vi "filter_calcs.vi"(8 "Detector 3 Correlations In":T1, 9 "Detector 1 Correlations In":T1, 10 "Detector 3":i16, 11 "Detector 1":i16) -> (0 "Detector 3 Correlations Out":T1, 1 "Detector 1 Correlations Out":T1)   [LabVIEW 2015]
uses:
  Detector_Cluster.ctl
  <vilib>/rvi/Emulation/niFpgaEmulationIsFPGAContextNoSignature.vi
  <vilib>/rvi/Emulation/niFpgaSctlEmulationGetInTimedLoop.vi
  <vilib>/rvi/errors/niFpgaSetErrorForExecOnDevCompSimple.vi
  <vilib>/rvi/eio/common/nirviEmuReportErrorAndStop.vi
  <vilib>/rvi/DataTransferAndStorage/Container/Common/niFpgaContainerGetUniqueNameForEmu.vi
  <vilib>/rvi/FIFO/Fifo_Resource/nirvififoEmulationSetSize.vi
  <vilib>/rvi/FIFO/Fifo_Resource/nirviFifoEmulationQueueMgr.vi
  <instcachedir>/0/nirviFifoEmulationQueueMgr_E5CAEC123FF24DC58D834DCA3CDAA9B5.lvgen/nirviFifoEmulationQueueMgr_E5CAEC123FF24DC58D834DCA3CDAA9B5_002.vi
  <vilib>/rvi/FIFO/Fifo_Resource/nirvififoEmulationDetermineInputValidOut.vi
  <vilib>/rvi/FIFO/Fifo_Resource/nirvififoEmulationCreateLock.vi
  <vilib>/rvi/Emulation/niFpgaProcessEmulError.vi
  <vilib>/rvi/FIFO/Fifo_Resource/nirvififoEmulationObtainLock.vi
  <vilib>/rvi/FIFO/Fifo_Resource/nirvififoEmulationReleaseLock.vi
  <vilib>/rvi/occurrence/nirviWaitOnOccurrenceBase.vi
  <vilib>/rvi/errors/nirviReportUnexpectedCaseInternalError.vi
  <vilib>/rvi/errors/nirviReportUnexpectedCaseInternalError (U32).vi
  <vilib>/rvi/DataTransferAndStorage/Container/Common/niFpgaContainerExecOnDevCompGetState.vi
  <vilib>/Utility/error.llb/Clear Errors.vi
  <vilib>/rvi/interface/RandomDataEmulation/niFpgaRandomDataHandleErrors.vi
  <vilib>/rvi/DataTransferAndStorage/Container/XNode/niFpgaContainer.xnode
  <vilib>/rvi/FIFO/Fifo_Resource/nirvififoEmulationWrite.vi
  <vilib>/rvi/FIFO/Fifo_Resource/niFpgaFifoEmulationRefIn.vi
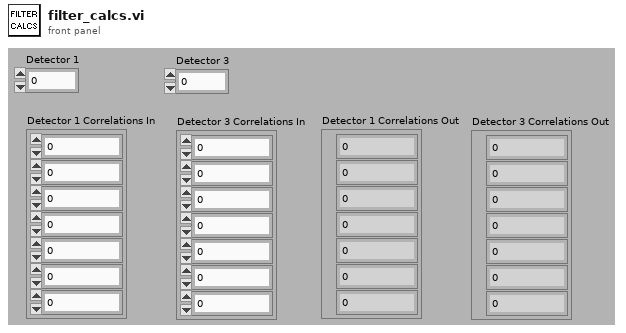
[diagram p1: front panel]
types:
  T1 = typedef "Detector_Cluster.ctl" = cluster{"1":i32, "2":i32, "3":i32, "4":i32, "5":i32, "6":i32, "7":i32}
  T2 = cluster{"Average Out":i32, "Next State":u16, "Detector 1 Correlation out":i32, "Detector 3 Correlation out":i32, "Velocity Count out":i32, "Detector counter out":i32, "Timeout count out":u32}
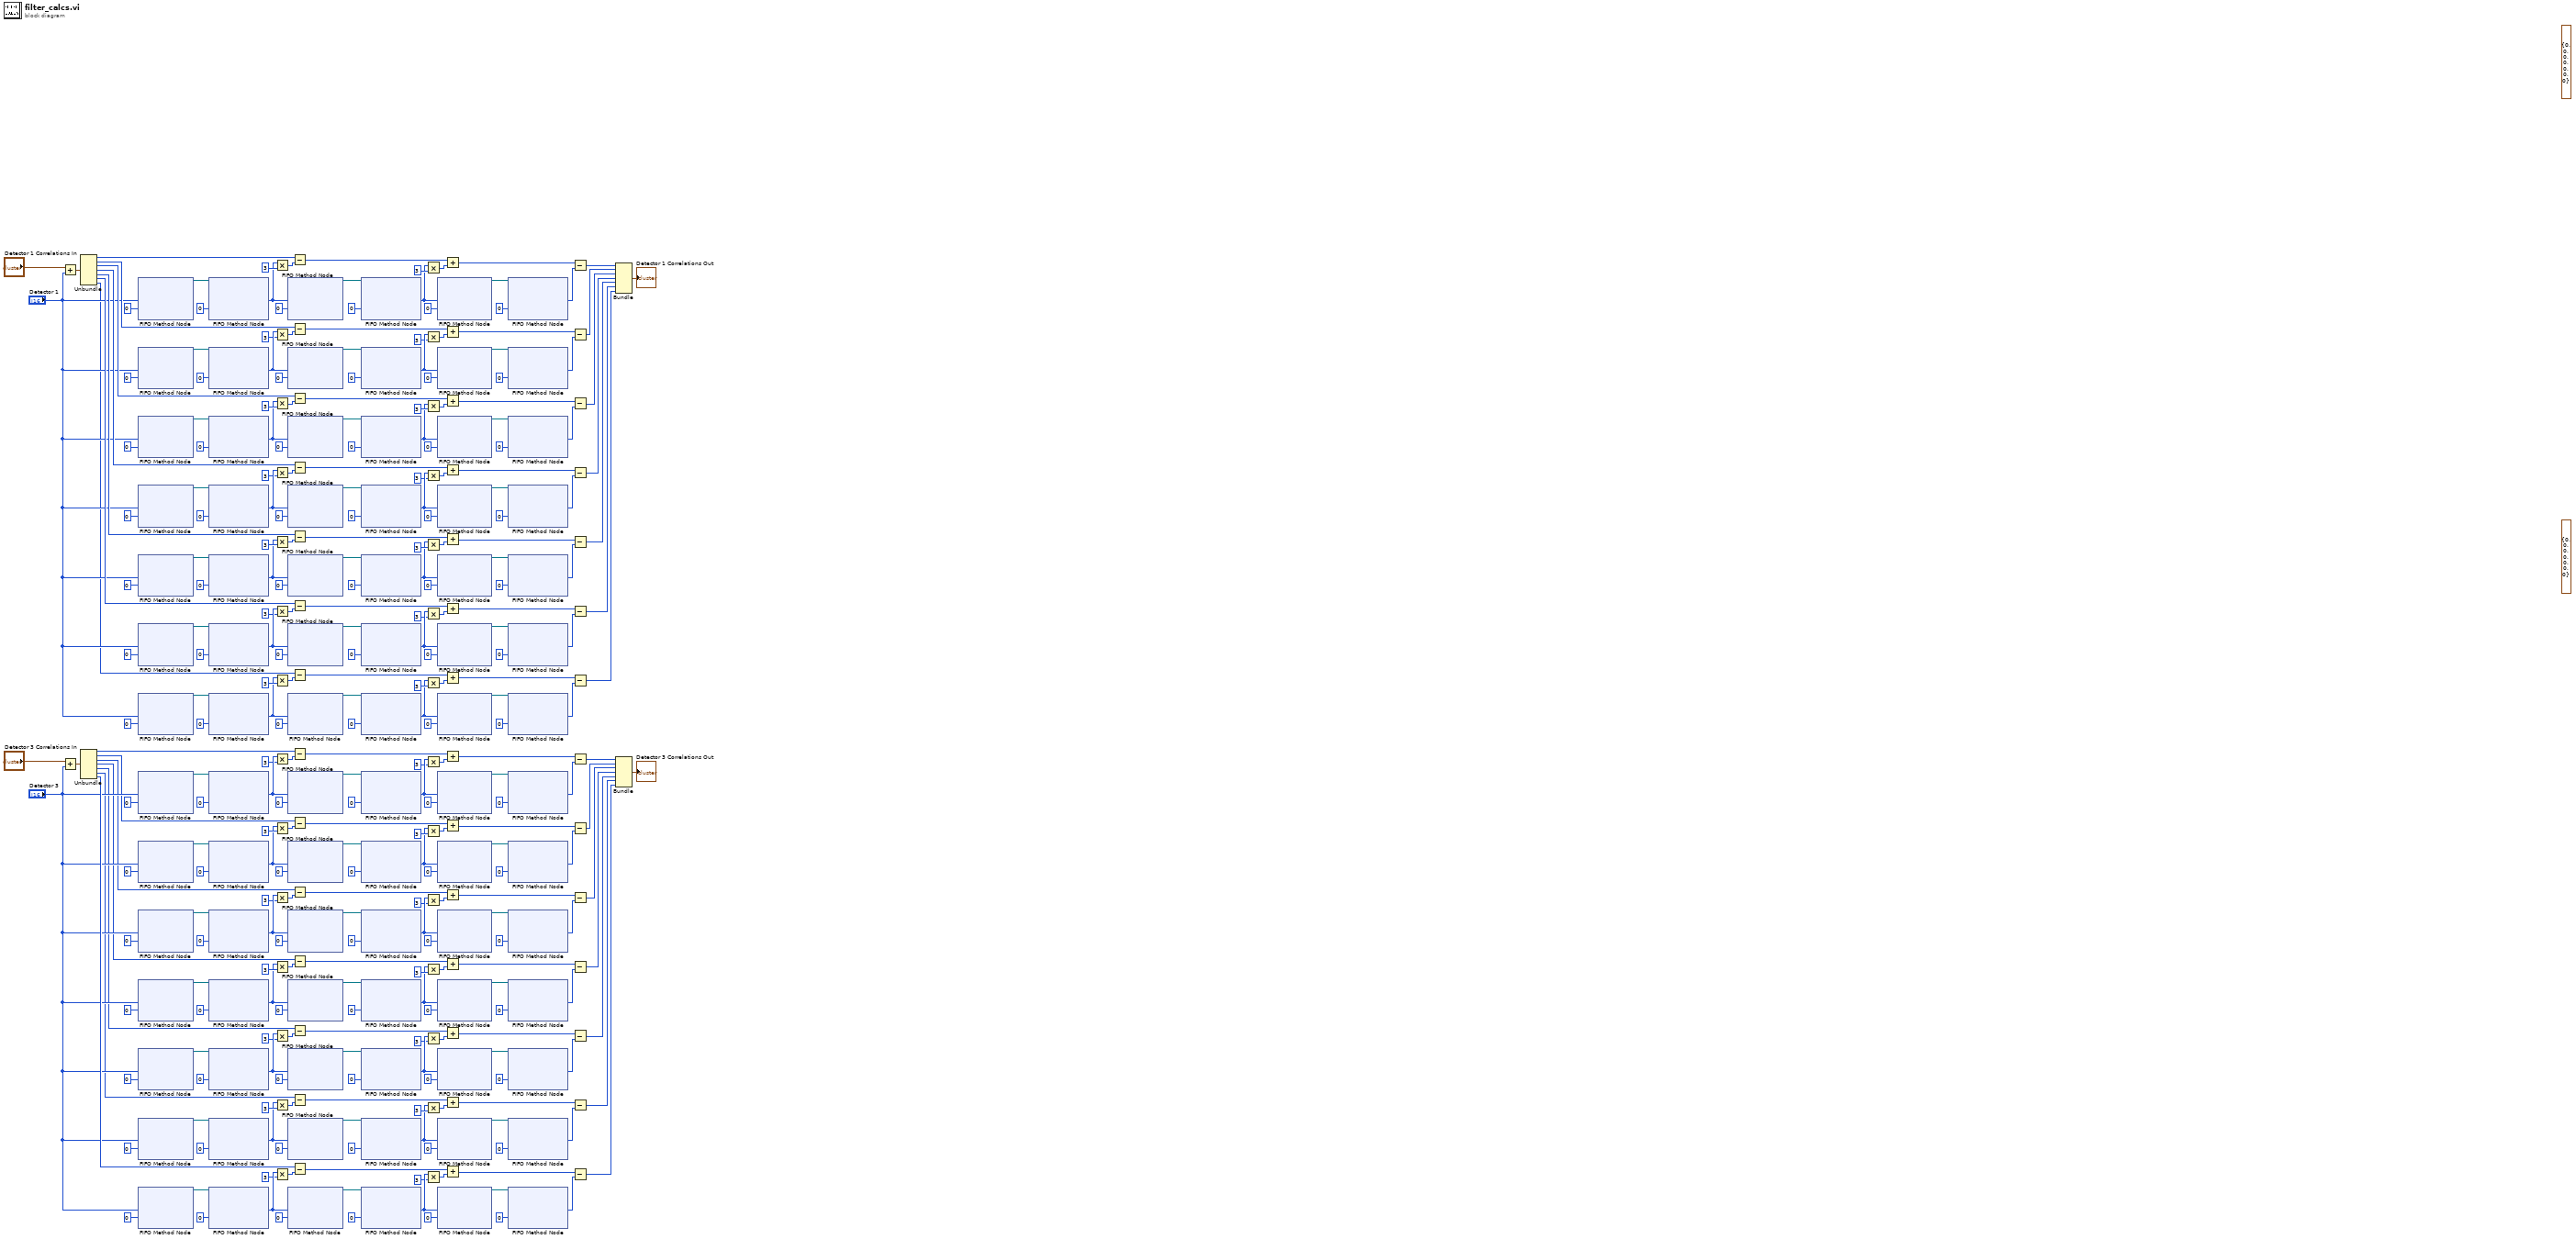
[diagram p0: block diagram]
diagram:
  (unwired) T2 {"Average Out"=0, "Next State"=0, "Detector 1 Correlation out"=0, "Detector 3 Correlation out"=0, "Velocity Count out"=0, "Detector counter out"=0, "Timeout count out"=0} ("Output Cluster")
  (unwired) T2 {"Average Out"=0, "Next State"=0, "Detector 1 Correlation out"=0, "Detector 3 Correlation out"=0, "Velocity Count out"=0, "Detector counter out"=0, "Timeout count out"=0} ("Output Cluster")
  n1 = Add(x="Detector 1 Correlations In", y="Detector 1") -> (x+y=w275:T1)
  n2 = Add(x="Detector 3 Correlations In", y="Detector 3") -> (x+y=w14:T1)
  n3 = Unbundle(w275) -> ("1"=w273:i32, "2"=w247:i32, "3"=w226:i32, "4"=w207:i32, "5"=w187:i32, "6"=w167:i32, "7"=w146:i32)
  n4 = Unbundle(w14) -> ("1"=w16:i32, "2"=w42:i32, "3"=w63:i32, "4"=w82:i32, "5"=w102:i32, "6"=w122:i32, "7"=w143:i32)
  n5 = xnode ("FIFO Method Node")("Element"="Detector 1", "Timeout"=0) -> ("FIFO Out"=w278:refnum<k21>)  [unwired: 1 in, 1 out]
  n6 = xnode ("FIFO Method Node")("Element"="Detector 1", "Timeout"=0) -> ("FIFO Out"=w258:refnum<k21>)  [unwired: 1 in, 1 out]
  n7 = xnode ("FIFO Method Node")("Element"="Detector 1", "Timeout"=0) -> ("FIFO Out"=w235:refnum<k21>)  [unwired: 1 in, 1 out]
  n8 = xnode ("FIFO Method Node")("Element"="Detector 1", "Timeout"=0) -> ("FIFO Out"=w218:refnum<k21>)  [unwired: 1 in, 1 out]
  n9 = xnode ("FIFO Method Node")("Element"="Detector 1", "Timeout"=0) -> ("FIFO Out"=w195:refnum<k21>)  [unwired: 1 in, 1 out]
  n10 = xnode ("FIFO Method Node")("Element"="Detector 1", "Timeout"=0) -> ("FIFO Out"=w178:refnum<k21>)  [unwired: 1 in, 1 out]
  n11 = xnode ("FIFO Method Node")("Element"="Detector 1", "Timeout"=0) -> ("FIFO Out"=w155:refnum<k21>)  [unwired: 1 in, 1 out]
  n12 = xnode ("FIFO Method Node")("Element"="Detector 3", "Timeout"=0) -> ("FIFO Out"=w11:refnum<k21>)  [unwired: 1 in, 1 out]
  n13 = xnode ("FIFO Method Node")("Element"="Detector 3", "Timeout"=0) -> ("FIFO Out"=w31:refnum<k21>)  [unwired: 1 in, 1 out]
  n14 = xnode ("FIFO Method Node")("Element"="Detector 3", "Timeout"=0) -> ("FIFO Out"=w54:refnum<k21>)  [unwired: 1 in, 1 out]
  n15 = xnode ("FIFO Method Node")("Element"="Detector 3", "Timeout"=0) -> ("FIFO Out"=w71:refnum<k21>)  [unwired: 1 in, 1 out]
  n16 = xnode ("FIFO Method Node")("Element"="Detector 3", "Timeout"=0) -> ("FIFO Out"=w94:refnum<k21>)  [unwired: 1 in, 1 out]
  n17 = xnode ("FIFO Method Node")("Element"="Detector 3", "Timeout"=0) -> ("FIFO Out"=w111:refnum<k21>)  [unwired: 1 in, 1 out]
  n18 = xnode ("FIFO Method Node")("Element"="Detector 3", "Timeout"=0) -> ("FIFO Out"=w134:refnum<k21>)  [unwired: 1 in, 1 out]
  n19 = xnode ("FIFO Method Node")("Timeout"=0, "FIFO In"=w278) -> ("Element"=w284:i16)  [unwired: 2 out]
  n20 = xnode ("FIFO Method Node")("Timeout"=0, "FIFO In"=w258) -> ("Element"=w252:i16)  [unwired: 2 out]
  n21 = xnode ("FIFO Method Node")("Timeout"=0, "FIFO In"=w235) -> ("Element"=w241:i16)  [unwired: 2 out]
  n22 = xnode ("FIFO Method Node")("Timeout"=0, "FIFO In"=w218) -> ("Element"=w212:i16)  [unwired: 2 out]
  n23 = xnode ("FIFO Method Node")("Timeout"=0, "FIFO In"=w195) -> ("Element"=w201:i16)  [unwired: 2 out]
  n24 = xnode ("FIFO Method Node")("Timeout"=0, "FIFO In"=w178) -> ("Element"=w172:i16)  [unwired: 2 out]
  n25 = xnode ("FIFO Method Node")("Timeout"=0, "FIFO In"=w155) -> ("Element"=w161:i16)  [unwired: 2 out]
  n26 = xnode ("FIFO Method Node")("Timeout"=0, "FIFO In"=w11) -> ("Element"=w5:i16)  [unwired: 2 out]
  n27 = xnode ("FIFO Method Node")("Timeout"=0, "FIFO In"=w31) -> ("Element"=w37:i16)  [unwired: 2 out]
  n28 = xnode ("FIFO Method Node")("Timeout"=0, "FIFO In"=w54) -> ("Element"=w48:i16)  [unwired: 2 out]
  n29 = xnode ("FIFO Method Node")("Timeout"=0, "FIFO In"=w71) -> ("Element"=w77:i16)  [unwired: 2 out]
  n30 = xnode ("FIFO Method Node")("Timeout"=0, "FIFO In"=w94) -> ("Element"=w88:i16)  [unwired: 2 out]
  n31 = xnode ("FIFO Method Node")("Timeout"=0, "FIFO In"=w111) -> ("Element"=w117:i16)  [unwired: 2 out]
  n32 = xnode ("FIFO Method Node")("Timeout"=0, "FIFO In"=w134) -> ("Element"=w128:i16)  [unwired: 2 out]
  n33 = Multiply(x=w284, y=i16 3) -> (x*y=w274:i16)
  n34 = Multiply(x=w252, y=i16 3) -> (x*y=w261:i16)
  n35 = Multiply(x=w241, y=i16 3) -> (x*y=w232:i16)
  n36 = Multiply(x=w212, y=i16 3) -> (x*y=w221:i16)
  n37 = Multiply(x=w201, y=i16 3) -> (x*y=w192:i16)
  n38 = Multiply(x=w172, y=i16 3) -> (x*y=w181:i16)
  n39 = Multiply(x=w161, y=i16 3) -> (x*y=w152:i16)
  n40 = Multiply(x=w5, y=i16 3) -> (x*y=w15:i16)
  n41 = Multiply(x=w37, y=i16 3) -> (x*y=w28:i16)
  n42 = Multiply(x=w48, y=i16 3) -> (x*y=w57:i16)
  n43 = Multiply(x=w77, y=i16 3) -> (x*y=w68:i16)
  n44 = Multiply(x=w88, y=i16 3) -> (x*y=w97:i16)
  n45 = Multiply(x=w117, y=i16 3) -> (x*y=w108:i16)
  n46 = Multiply(x=w128, y=i16 3) -> (x*y=w137:i16)
  n47 = xnode ("FIFO Method Node")("Element"=w284, "Timeout"=0) -> ("FIFO Out"=w277:refnum<k21>)  [unwired: 1 in, 1 out]
  n48 = xnode ("FIFO Method Node")("Element"=w252, "Timeout"=0) -> ("FIFO Out"=w259:refnum<k21>)  [unwired: 1 in, 1 out]
  n49 = xnode ("FIFO Method Node")("Element"=w241, "Timeout"=0) -> ("FIFO Out"=w234:refnum<k21>)  [unwired: 1 in, 1 out]
  n50 = xnode ("FIFO Method Node")("Element"=w212, "Timeout"=0) -> ("FIFO Out"=w219:refnum<k21>)  [unwired: 1 in, 1 out]
  n51 = xnode ("FIFO Method Node")("Element"=w201, "Timeout"=0) -> ("FIFO Out"=w194:refnum<k21>)  [unwired: 1 in, 1 out]
  n52 = xnode ("FIFO Method Node")("Element"=w172, "Timeout"=0) -> ("FIFO Out"=w179:refnum<k21>)  [unwired: 1 in, 1 out]
  n53 = xnode ("FIFO Method Node")("Element"=w161, "Timeout"=0) -> ("FIFO Out"=w154:refnum<k21>)  [unwired: 1 in, 1 out]
  n54 = xnode ("FIFO Method Node")("Element"=w5, "Timeout"=0) -> ("FIFO Out"=w12:refnum<k21>)  [unwired: 1 in, 1 out]
  n55 = xnode ("FIFO Method Node")("Element"=w37, "Timeout"=0) -> ("FIFO Out"=w30:refnum<k21>)  [unwired: 1 in, 1 out]
  n56 = xnode ("FIFO Method Node")("Element"=w48, "Timeout"=0) -> ("FIFO Out"=w55:refnum<k21>)  [unwired: 1 in, 1 out]
  n57 = xnode ("FIFO Method Node")("Element"=w77, "Timeout"=0) -> ("FIFO Out"=w70:refnum<k21>)  [unwired: 1 in, 1 out]
  n58 = xnode ("FIFO Method Node")("Element"=w88, "Timeout"=0) -> ("FIFO Out"=w95:refnum<k21>)  [unwired: 1 in, 1 out]
  n59 = xnode ("FIFO Method Node")("Element"=w117, "Timeout"=0) -> ("FIFO Out"=w110:refnum<k21>)  [unwired: 1 in, 1 out]
  n60 = xnode ("FIFO Method Node")("Element"=w128, "Timeout"=0) -> ("FIFO Out"=w135:refnum<k21>)  [unwired: 1 in, 1 out]
  n61 = Subtract(x=w273, y=w274) -> (x-y=w267:i32)
  n62 = Subtract(x=w247, y=w261) -> (x-y=w265:i32)
  n63 = Subtract(x=w226, y=w232) -> (x-y=w228:i32)
  n64 = Subtract(x=w207, y=w221) -> (x-y=w225:i32)
  n65 = Subtract(x=w187, y=w192) -> (x-y=w188:i32)
  n66 = Subtract(x=w167, y=w181) -> (x-y=w185:i32)
  n67 = Subtract(x=w146, y=w152) -> (x-y=w148:i32)
  n68 = Subtract(x=w16, y=w15) -> (x-y=w22:i32)
  n69 = Subtract(x=w42, y=w28) -> (x-y=w24:i32)
  n70 = Subtract(x=w63, y=w57) -> (x-y=w61:i32)
  n71 = Subtract(x=w82, y=w68) -> (x-y=w64:i32)
  n72 = Subtract(x=w102, y=w97) -> (x-y=w101:i32)
  n73 = Subtract(x=w122, y=w108) -> (x-y=w104:i32)
  n74 = Subtract(x=w143, y=w137) -> (x-y=w141:i32)
  n75 = xnode ("FIFO Method Node")("Timeout"=0, "FIFO In"=w277) -> ("Element"=w280:i16)  [unwired: 2 out]
  n76 = xnode ("FIFO Method Node")("Timeout"=0, "FIFO In"=w259) -> ("Element"=w256:i16)  [unwired: 2 out]
  n77 = xnode ("FIFO Method Node")("Timeout"=0, "FIFO In"=w234) -> ("Element"=w237:i16)  [unwired: 2 out]
  n78 = xnode ("FIFO Method Node")("Timeout"=0, "FIFO In"=w219) -> ("Element"=w216:i16)  [unwired: 2 out]
  n79 = xnode ("FIFO Method Node")("Timeout"=0, "FIFO In"=w194) -> ("Element"=w197:i16)  [unwired: 2 out]
  n80 = xnode ("FIFO Method Node")("Timeout"=0, "FIFO In"=w179) -> ("Element"=w176:i16)  [unwired: 2 out]
  n81 = xnode ("FIFO Method Node")("Timeout"=0, "FIFO In"=w154) -> ("Element"=w157:i16)  [unwired: 2 out]
  n82 = xnode ("FIFO Method Node")("Timeout"=0, "FIFO In"=w12) -> ("Element"=w9:i16)  [unwired: 2 out]
  n83 = xnode ("FIFO Method Node")("Timeout"=0, "FIFO In"=w30) -> ("Element"=w33:i16)  [unwired: 2 out]
  n84 = xnode ("FIFO Method Node")("Timeout"=0, "FIFO In"=w55) -> ("Element"=w52:i16)  [unwired: 2 out]
  n85 = xnode ("FIFO Method Node")("Timeout"=0, "FIFO In"=w70) -> ("Element"=w73:i16)  [unwired: 2 out]
  n86 = xnode ("FIFO Method Node")("Timeout"=0, "FIFO In"=w95) -> ("Element"=w92:i16)  [unwired: 2 out]
  n87 = xnode ("FIFO Method Node")("Timeout"=0, "FIFO In"=w110) -> ("Element"=w113:i16)  [unwired: 2 out]
  n88 = xnode ("FIFO Method Node")("Timeout"=0, "FIFO In"=w135) -> ("Element"=w132:i16)  [unwired: 2 out]
  n89 = Multiply(x=w280, y=i16 3) -> (x*y=w268:i16)
  n90 = Multiply(x=w256, y=i16 3) -> (x*y=w264:i16)
  n91 = Multiply(x=w237, y=i16 3) -> (x*y=w229:i16)
  n92 = Multiply(x=w216, y=i16 3) -> (x*y=w224:i16)
  n93 = Multiply(x=w197, y=i16 3) -> (x*y=w189:i16)
  n94 = Multiply(x=w176, y=i16 3) -> (x*y=w184:i16)
  n95 = Multiply(x=w157, y=i16 3) -> (x*y=w149:i16)
  n96 = Multiply(x=w9, y=i16 3) -> (x*y=w21:i16)
  n97 = Multiply(x=w33, y=i16 3) -> (x*y=w25:i16)
  n98 = Multiply(x=w52, y=i16 3) -> (x*y=w60:i16)
  n99 = Multiply(x=w73, y=i16 3) -> (x*y=w65:i16)
  n100 = Multiply(x=w92, y=i16 3) -> (x*y=w100:i16)
  n101 = Multiply(x=w113, y=i16 3) -> (x*y=w105:i16)
  n102 = Multiply(x=w132, y=i16 3) -> (x*y=w140:i16)
  n103 = xnode ("FIFO Method Node")("Element"=w280, "Timeout"=0) -> ("FIFO Out"=w276:refnum<k21>)  [unwired: 1 in, 1 out]
  n104 = xnode ("FIFO Method Node")("Element"=w256, "Timeout"=0) -> ("FIFO Out"=w260:refnum<k21>)  [unwired: 1 in, 1 out]
  n105 = xnode ("FIFO Method Node")("Element"=w237, "Timeout"=0) -> ("FIFO Out"=w233:refnum<k21>)  [unwired: 1 in, 1 out]
  n106 = xnode ("FIFO Method Node")("Element"=w216, "Timeout"=0) -> ("FIFO Out"=w220:refnum<k21>)  [unwired: 1 in, 1 out]
  n107 = xnode ("FIFO Method Node")("Element"=w197, "Timeout"=0) -> ("FIFO Out"=w193:refnum<k21>)  [unwired: 1 in, 1 out]
  n108 = xnode ("FIFO Method Node")("Element"=w176, "Timeout"=0) -> ("FIFO Out"=w180:refnum<k21>)  [unwired: 1 in, 1 out]
  n109 = xnode ("FIFO Method Node")("Element"=w157, "Timeout"=0) -> ("FIFO Out"=w153:refnum<k21>)  [unwired: 1 in, 1 out]
  n110 = xnode ("FIFO Method Node")("Element"=w9, "Timeout"=0) -> ("FIFO Out"=w13:refnum<k21>)  [unwired: 1 in, 1 out]
  n111 = xnode ("FIFO Method Node")("Element"=w33, "Timeout"=0) -> ("FIFO Out"=w29:refnum<k21>)  [unwired: 1 in, 1 out]
  n112 = xnode ("FIFO Method Node")("Element"=w52, "Timeout"=0) -> ("FIFO Out"=w56:refnum<k21>)  [unwired: 1 in, 1 out]
  n113 = xnode ("FIFO Method Node")("Element"=w73, "Timeout"=0) -> ("FIFO Out"=w69:refnum<k21>)  [unwired: 1 in, 1 out]
  n114 = xnode ("FIFO Method Node")("Element"=w92, "Timeout"=0) -> ("FIFO Out"=w96:refnum<k21>)  [unwired: 1 in, 1 out]
  n115 = xnode ("FIFO Method Node")("Element"=w113, "Timeout"=0) -> ("FIFO Out"=w109:refnum<k21>)  [unwired: 1 in, 1 out]
  n116 = xnode ("FIFO Method Node")("Element"=w132, "Timeout"=0) -> ("FIFO Out"=w136:refnum<k21>)  [unwired: 1 in, 1 out]
  n117 = Add(x=w267, y=w268) -> (x+y=w272:i32)
  n118 = Add(x=w265, y=w264) -> (x+y=w262:i32)
  n119 = Add(x=w228, y=w229) -> (x+y=w231:i32)
  n120 = Add(x=w225, y=w224) -> (x+y=w222:i32)
  n121 = Add(x=w188, y=w189) -> (x+y=w191:i32)
  n122 = Add(x=w185, y=w184) -> (x+y=w182:i32)
  n123 = Add(x=w148, y=w149) -> (x+y=w151:i32)
  n124 = Add(x=w22, y=w21) -> (x+y=w17:i32)
  n125 = Add(x=w24, y=w25) -> (x+y=w27:i32)
  n126 = Add(x=w61, y=w60) -> (x+y=w58:i32)
  n127 = Add(x=w64, y=w65) -> (x+y=w67:i32)
  n128 = Add(x=w101, y=w100) -> (x+y=w98:i32)
  n129 = Add(x=w104, y=w105) -> (x+y=w107:i32)
  n130 = Add(x=w141, y=w140) -> (x+y=w138:i32)
  n131 = xnode ("FIFO Method Node")("Timeout"=0, "FIFO In"=w276) -> ("Element"=w270:i16)  [unwired: 2 out]
  n132 = xnode ("FIFO Method Node")("Timeout"=0, "FIFO In"=w260) -> ("Element"=w263:i16)  [unwired: 2 out]
  n133 = xnode ("FIFO Method Node")("Timeout"=0, "FIFO In"=w233) -> ("Element"=w230:i16)  [unwired: 2 out]
  n134 = xnode ("FIFO Method Node")("Timeout"=0, "FIFO In"=w220) -> ("Element"=w223:i16)  [unwired: 2 out]
  n135 = xnode ("FIFO Method Node")("Timeout"=0, "FIFO In"=w193) -> ("Element"=w190:i16)  [unwired: 2 out]
  n136 = xnode ("FIFO Method Node")("Timeout"=0, "FIFO In"=w180) -> ("Element"=w183:i16)  [unwired: 2 out]
  n137 = xnode ("FIFO Method Node")("Timeout"=0, "FIFO In"=w153) -> ("Element"=w150:i16)  [unwired: 2 out]
  n138 = xnode ("FIFO Method Node")("Timeout"=0, "FIFO In"=w13) -> ("Element"=w19:i16)  [unwired: 2 out]
  n139 = xnode ("FIFO Method Node")("Timeout"=0, "FIFO In"=w29) -> ("Element"=w26:i16)  [unwired: 2 out]
  n140 = xnode ("FIFO Method Node")("Timeout"=0, "FIFO In"=w56) -> ("Element"=w59:i16)  [unwired: 2 out]
  n141 = xnode ("FIFO Method Node")("Timeout"=0, "FIFO In"=w69) -> ("Element"=w66:i16)  [unwired: 2 out]
  n142 = xnode ("FIFO Method Node")("Timeout"=0, "FIFO In"=w96) -> ("Element"=w99:i16)  [unwired: 2 out]
  n143 = xnode ("FIFO Method Node")("Timeout"=0, "FIFO In"=w109) -> ("Element"=w106:i16)  [unwired: 2 out]
  n144 = xnode ("FIFO Method Node")("Timeout"=0, "FIFO In"=w136) -> ("Element"=w139:i16)  [unwired: 2 out]
  n145 = Subtract(x=w272, y=w270) -> (x-y=w271:i32)
  n146 = Subtract(x=w262, y=w263) -> (x-y=w246:i32)
  n147 = Subtract(x=w231, y=w230) -> (x-y=w227:i32)
  n148 = Subtract(x=w222, y=w223) -> (x-y=w206:i32)
  n149 = Subtract(x=w191, y=w190) -> (x-y=w186:i32)
  n150 = Subtract(x=w182, y=w183) -> (x-y=w166:i32)
  n151 = Subtract(x=w151, y=w150) -> (x-y=w145:i32)
  n152 = Subtract(x=w17, y=w19) -> (x-y=w18:i32)
  n153 = Subtract(x=w27, y=w26) -> (x-y=w43:i32)
  n154 = Subtract(x=w58, y=w59) -> (x-y=w62:i32)
  n155 = Subtract(x=w67, y=w66) -> (x-y=w83:i32)
  n156 = Subtract(x=w98, y=w99) -> (x-y=w103:i32)
  n157 = Subtract(x=w107, y=w106) -> (x-y=w123:i32)
  n158 = Subtract(x=w138, y=w139) -> (x-y=w144:i32)
  n159 = Bundle(w271, w246, w227, w206, w186, w166, w145) -> (→"Detector 1 Correlations Out":cluster{i32, i32, i32, i32, i32, i32, i32})  [unwired: 1 in]
  n160 = Bundle(w18, w43, w62, w83, w103, w123, w144) -> (→"Detector 3 Correlations Out":cluster{i32, i32, i32, i32, i32, i32, i32})  [unwired: 1 in]
